vi "Simulation iRobot Open.vi"(8 "error in (no error)":errorcluster) -> (0 "error out":errorcluster, 2 "initial position":sgl[](array[numeric]), 3 "simulator":T1={"configuration"={"maxTime"=5.0, "enableVisualization"=TRUE, "statechart"=path "iRobot Navigation State Machine.vi", "environment"=path "simulation configuration.ini", "record"=path "Simulation Record.xml", "autograde?"=TRUE, "interactive?"=FALSE, "feedback mode"=enum."debug navigation"}, "Bump Sensors"=[], "Distance Sensors"=[], "Accelerometer"=refnum, "Wall Sensor"=refnum, "Statechart\ndisplay"=refnum, "Body"=refnum, "Left Motor"=refnum, "Right Motor"=refnum, "first step?"=FALSE})   [LabVIEW 2013]
doc: "Begins a simulation of the Cal Climber."
uses:
  Simulator.ctl
  <instrlib>/DC Motor Controller/HAIOL/DC Motor Controller.lvclass
  CyberSim interface/Simulation Configuration.ctl
  autograder/feedbackMode.ctl
  <vilib>/robotics/Simulator/Engine/ctl/DeviceID.ctl
  <vilib>/robotics/Simulator/Interface/Simulator References/Get Robot Body Reference.vi
  <vilib>/robotics/Simulator/Interface/Simulator References/Get Sensor Reference.vi
  <vilib>/robotics/Simulator/NI_Robotics_Simulator.lvlib
  <resource>/objmgr/LVODE.rc
  <instrlib>/DC Motor Controller/HAIOL/Simulator/DC Motor Controller Simulator.lvclass
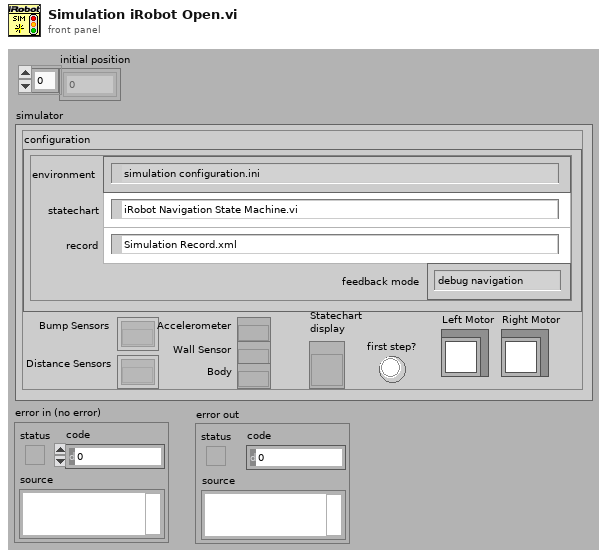
[diagram p1: front panel]
types:
  T1 = typedef "Simulator.ctl" = cluster{"configuration":T2, "Bump Sensors":refnum<k20>[], "Distance Sensors":refnum<k20>[], "Accelerometer":refnum<k20>, "Wall Sensor":refnum<k20>, "Statechart\ndisplay":refnum<vi>, "Body":refnum<k20>, "Left Motor":refnum<class "DC Motor Controller.lvclass">, "Right Motor":refnum<class "DC Motor Controller.lvclass">, "first step?":bool}
  T2 = typedef "Simulation Configuration.ctl" = cluster{"maxTime":sgl, "enableVisualization":bool, "statechart":path, "environment":path, "record":path, "autograde?":bool, "interactive?":bool, "feedback mode":T3}
  T3 = typedef "feedbackMode.ctl" = enum32{"debug navigation", "debug hill climb", "autograde navigation", "autograde hill climb"}
  T4 = typedef "NI_Robotics_Simulator.lvlib/DeviceID.ctl" = cluster{"robot ID":string, "sensor/actuator ID":string}
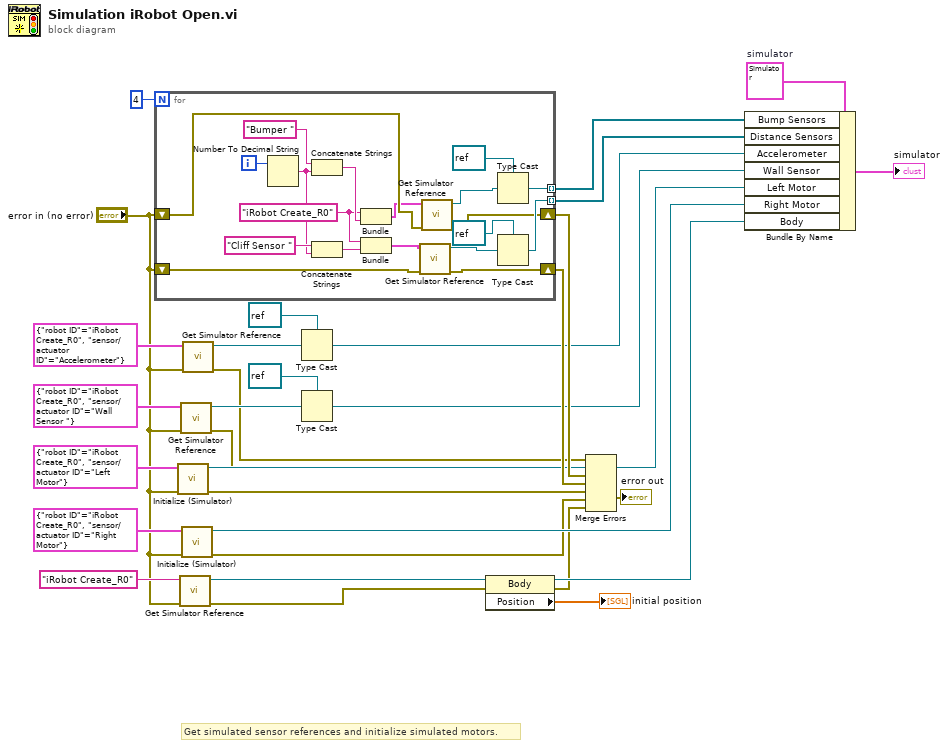
[diagram p0: block diagram]
diagram:
  w24 = T1 {"configuration"={"maxTime"=0.0, "enableVisualization"=FALSE, "statechart"=path "", "environment"=path "", "record"=path "", "autograde?"=FALSE, "interactive?"=FALSE, "feedback mode"=enum."debug navigation"}, "Bump Sensors"=[], "Distance Sensors"=[], "Accelerometer"=refnum, "Wall Sensor"=refnum, "Statechart\ndisplay"=refnum, "Body"=refnum, "Left Motor"=refnum, "Right Motor"=refnum, "first step?"=FALSE}  # simulator
  # "Get simulated sensor references and initialize simulated motors."
  n1 = for {
    N: 4 -> [_]
    tunnel: [w47] -> w25 mode=indexing
    tunnel: [w41] -> w26 mode=indexing
    shift-right: [w36] -> w27
    shift-left: "error in (no error)" -> [w39]
    shift-right: [w33] -> w28
    shift-left: "error in (no error)" -> [w34]
    i -> [w50]
    w40 = "iRobot Create_R0" ("Robot ID")
    n2 = Number To Decimal String(number=w50) -> (decimal integer string=w44:string)  [unwired: 1 in]
    n3 = Concatenate Strings("Bumper " ("Device Label"), w44) -> (w43:string)
    n4 = Concatenate Strings("Cliff Sensor " ("Device Label"), w44) -> (w48:string)
    n5 = Bundle("Robot ID"=w40, w43) -> (w38:cluster{"Robot ID":string, string})  [unwired: 1 in]
    n6 = Bundle("Robot ID"=w40, w48) -> (w35:cluster{"Robot ID":string, string})  [unwired: 1 in]
    n7 = call-poly <vilib>:"Get Simulator Reference.vi"("error in (no error)"=w34, "device ID"=w35) -> ("error out"=w33:errorcluster, "sensor ref"=w32:refnum<k20>)  [unwired: 8 in]
    n8 = call-poly <vilib>:"Get Simulator Reference.vi"("error in (no error)"=w39, "device ID"=w38) -> ("error out"=w36:errorcluster, "sensor ref"=w37:refnum<k20>)  [unwired: 8 in]
    n9 = Type Cast(type=refnum<k20> refnum ("DistanceSensor Out"), x=w37) -> (*(type *) &x=w41:refnum<k20>)
    n10 = Type Cast(type=refnum<k20> refnum ("DistanceSensor Out"), x=w32) -> (*(type *) &x=w47:refnum<k20>)
  }
  n11 = call <instrlib>:"Initialize (Simulator).vi"("error in (no error)"="error in (no error)", "Device ID"=T4 {"robot ID"="iRobot Create_R0", "sensor/actuator ID"="Left Motor"}) -> ("error out"=w11:errorcluster, "DC Motor Controller out"=w12:refnum<class "DC Motor Controller.lvclass">)  [unwired: 8 in]
  n12 = call-poly <vilib>:"Get Simulator Reference.vi"("error in (no error)"="error in (no error)", "robot ID"="iRobot Create_R0" ("Robot ID")) -> ("error out"=w5:errorcluster, "robot body ref"=w6:refnum<k20>)  [unwired: 8 in]
  n13 = call-poly <vilib>:"Get Simulator Reference.vi"("error in (no error)"="error in (no error)", "device ID"=T4 {"robot ID"="iRobot Create_R0", "sensor/actuator ID"="Wall Sensor "} ("Device ID")) -> ("error out"=w4:errorcluster, "sensor ref"=w14:refnum<k20>)  [unwired: 8 in]
  n14 = call <instrlib>:"Initialize (Simulator).vi"("error in (no error)"="error in (no error)", "Device ID"=T4 {"robot ID"="iRobot Create_R0", "sensor/actuator ID"="Right Motor"}) -> ("error out"=w8:errorcluster, "DC Motor Controller out"=w9:refnum<class "DC Motor Controller.lvclass">)  [unwired: 8 in]
  n15 = call-poly <vilib>:"Get Simulator Reference.vi"("error in (no error)"="error in (no error)", "device ID"=T4 {"robot ID"="iRobot Create_R0", "sensor/actuator ID"="Accelerometer"} ("Device ID")) -> ("error out"=w3:errorcluster, "sensor ref"=w16:refnum<k20>)  [unwired: 8 in]
  n16 = Type Cast(type=refnum<k20> refnum ("DistanceSensor Out"), x=w16) -> (*(type *) &x=w23:refnum<k20>)
  n17 = Type Cast(type=refnum<k20> refnum ("DistanceSensor Out"), x=w14) -> (*(type *) &x=w22:refnum<k20>)
  n18 = property class="Body"(reference=w6, error in=w5) -> (reference out=w21:refnum<k20>, error out=w1:errorcluster, "Position"=→"initial position":sgl[])
  n19 = Merge Errors(w3, w4, w27, w28, w11, w8, w1) -> (→"error out":errorcluster)
  n20 = Bundle By Name(cluster=w24, "Bump Sensors"=w26, "Distance Sensors"=w25, "Accelerometer"=w23, "Wall Sensor"=w22, "Left Motor"=w12, "Right Motor"=w9, "Body"=w21) -> (→"simulator":T1)
